vi "Elevator.vi"(10 "Boolean":bool, 11 "Boolean 2":bool) -> (3 "Numeric":i32)   [LabVIEW 2017]
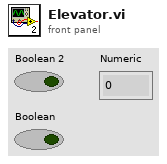
[diagram p1: front panel]
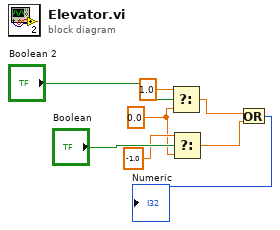
[diagram p0: block diagram]
diagram:
  w1 = 0.0 ("t")
  n1 = Select(t=1.0, s="Boolean 2", f=w1) -> (s? t:f=w6:dbl)
  n2 = Select(t=-1.0, s="Boolean", f=w1) -> (s? t:f=w7:dbl)
  n3 = Or(x=w6, y=w7) -> (x .or. y?=→"Numeric":i32)
